vi "dfd_Decide Processing Method.vi"(10 "order":i32=39, 11 "band counts":i32=4) -> (3 "processing method":T1=enum."Cosine-Modulated")   [LabVIEW 2017, in "NI_DigFilter_FilterBank.lvlib"]
uses:
  <vilib>/addons/Digital Filter Design/NI_DigFilter_FilterBank.lvlib
  <vilib>/addons/Digital Filter Design/FilterBank.llb/Object/DFD Filter Bank Processing Method.ctl
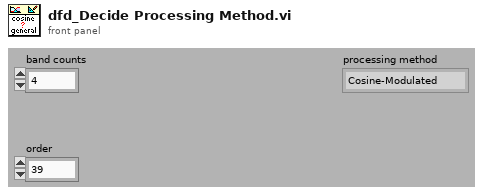
[diagram p1: front panel]
types:
  T1 = typedef "NI_DigFilter_FilterBank.lvlib/DFD Filter Bank Processing Method.ctl" = enum16{"General", "2-Band QMF Lattice", "Cosine-Modulated"}
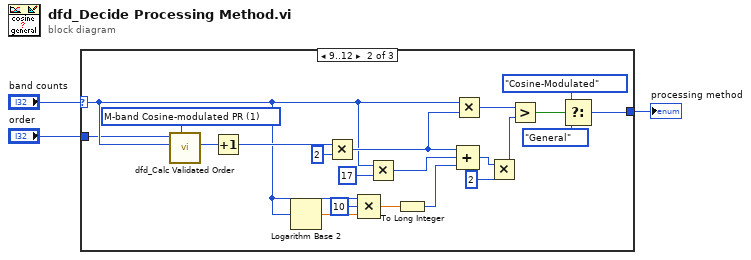
[diagram p0: block diagram]
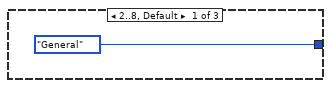
[diagram p2: hidden frame]
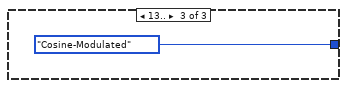
[diagram p3: hidden frame]
diagram:
  n1 = case shown="9..12" "band counts" {
    selector: "band counts" -> [_ w8 _]
    tunnel: [DFD_Filter_Bank_Processing_Method."General" ("f") w23 DFD_Filter_Bank_Processing_Method."Cosine-Modulated" ("processing method")] -> w3
    tunnel: "order" -> [_ w6 _]
    frame 2..8, Default {
    }
    frame 9..12 {
      w7 = u16 1 items=["2-band", "M-band Cosine-modulated PR"] ("bank type")
      n2 = call <vilib>:"dfd_Calc Validated Order.vi"("bank type"=w7, "bank counts"=w8, "order"=w6) -> ("validated order"=w5:i32)  [unwired: 6 in, 2 out]
      n3 = Increment(x=w5) -> (x+1=w22:i32)
      n4 = Logarithm Base 2(1:w8) -> (0:w19:dbl)
      n5 = Multiply(x=w22, y=2 ("value")) -> (x*y=w14:i32)
      n6 = Compound Arithmetic op=MULTIPLY(w8, 10 ("value"), w19) -> (w17:dbl)
      n7 = Multiply(x=w8, y=17 ("x")) -> (x*y=w15:i32)
      n8 = To Long Integer(number=w17) -> (32bit integer=w16:i32)
      n9 = Multiply(x=w8, y=w14) -> (x*y=w13:i32)
      n10 = Compound Arithmetic op=ADD(w14, w15, w16) -> (w11:i32)
      n11 = Multiply(x=w11, y=2) -> (x*y=w9:i32)
      n12 = Greater?(x=w13, y=w9) -> (0:w12:bool)
      n13 = Select(t=DFD_Filter_Bank_Processing_Method."Cosine-Modulated" ("processing method"), s=w12, f=DFD_Filter_Bank_Processing_Method."General") -> (s? t:f=w23:T1)
    }
    frame 13.. {
    }
  }
  "processing method" <- w3
